vi "PointMap_Duplicate.vi"(8 "error in (no error)":errorcluster, 10 "Source Map Name":string) -> (0 "error out":errorcluster, 3 "Map Out":T1)   [LabVIEW 2017, in "PointValueMap.lvlib"]
doc: "Copy one maps contents into another map. The destination map is created and will have the exact same contents as the source map."
uses:
  <vilib>/addons/PointValueMap/PointValueMap.lvlib
  <vilib>/addons/PointValueMap/controls/PointMap.ctl
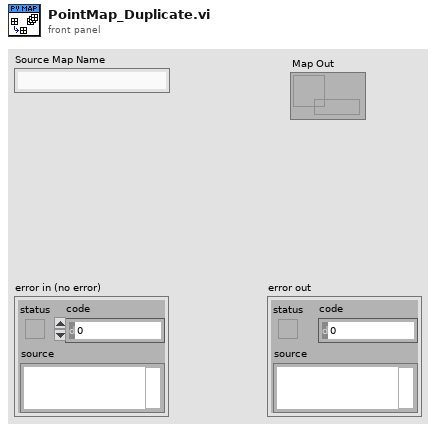
[diagram p1: front panel]
types:
  T1 = typedef "PointValueMap.lvlib/PointMap.ctl" = refnum<data-value>
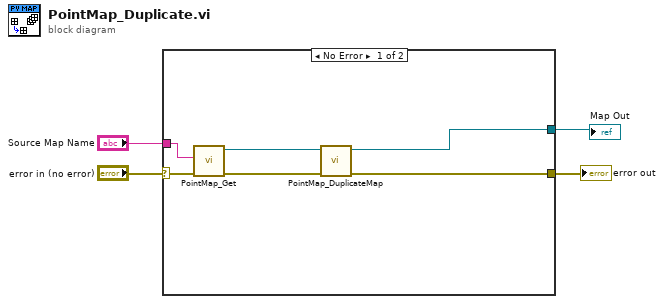
[diagram p0: block diagram]
diagram:
  n1 = case shown="No Error" "error in (no error)" {
    selector: "error in (no error)" -> [w9 w11]
    tunnel: "Source Map Name" -> [w10 _]
    tunnel: [w5 w11] -> w3
    tunnel: [w8 _] -> w1
    frame No Error {
      n2 = call <vilib>:"PointMap_Get.vi"("error in (no error)"=w9, "Name"=w10) -> ("error out"=w7:errorcluster, "Map Out"=w6:T1)  [unwired: 7 in, 1 out]
      n3 = call <vilib>:"PointMap_DuplicateMap.vi"("error in (no error)"=w7, "map in"=w6) -> ("error out"=w5:errorcluster, "duplicate map"=w8:T1)  [unwired: 8 in]
    }
    frame Error {
    }
  }
  "error out" <- w3
  "Map Out" <- w1
